vi "Workshop Exercise 2.vi"() -> ()   [LabVIEW 2019]
panel:
  in  "Enqueue Speed [ms]":u32=100
  in  "Dequeue Speed [ms]":u32=100
  out "Received Elements":dbl(graph)
  out "Generated Elements":dbl(graph)
  out "Elements in Queue":i32(slide) scale=0.0..100.0
  in  "Stop":bool
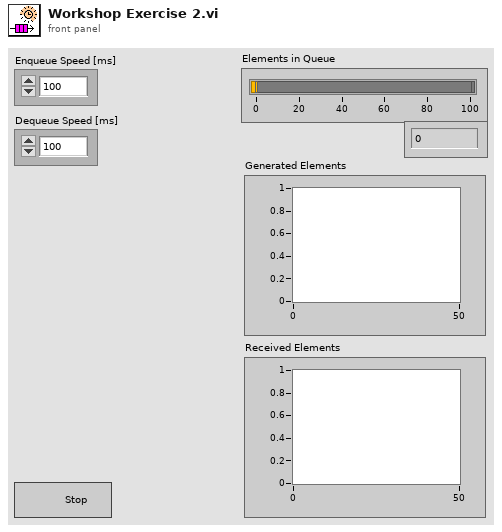
[diagram p1: front panel]
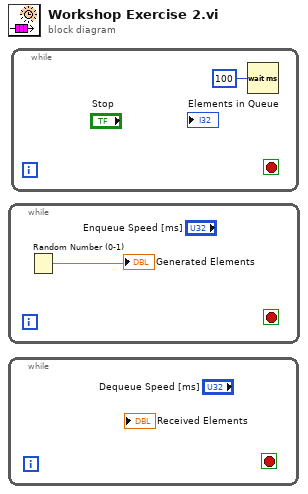
[diagram p0: block diagram]
diagram:
  n1 = while {
    stop <- _ stop-if-true
    # "Enqueue Loop"
    n2 = Random Number (0-1)() -> (number: 0 to 1=→"Generated Elements":dbl)
  }
  n3 = while {
    stop <- _ stop-if-true
    # "Dequeue Loop"
  }
  n4 = while {
    stop <- _ stop-if-true
    # "Queue Status"
    n5 = Wait (ms)(milliseconds to wait=u32 100) -> ()  [unwired: 1 out]
  }
